vi "FT_Write_String_Data_64bit.vi"(4 "error in (no error)":errorcluster, 6 "Buffer":string, 7 "Handle":u64) -> (0 "error out":errorcluster, 1 "FT_Status":u32(ring) items=["FT_OK", "FT_INVALID_HANDLE", "FT_DEVICE_NOT_FOUND", "FT_DEVICE_NOT_OPENED", "FT_IO_ERROR", "FT_INSUFFICIENT_RESOURCES", "FT_INVALID_PARAMETER", "FT_INVALID_BAUD_RATE", "FT_DEVICE_NOT_OPENED_FOR_ERASE", "FT_DEVICE_NOT_OPENED_FOR_WRITE", "FT_FAILED_TO_WRITE_DEVICE", "FT_EEPROM_READ_FAILED", "FT_EEPROM_WRITE_FAILED", "FT_EEPROM_ERASE_FAILED", "FT_EEPROM_NOT_PRESENT", "FT_EEPROM_NOT_PROGRAMMED", "FT_INVALID_ARGS", "FT_NOT_SUPPORTED", "FT_OTHER_ERROR"], 2 "Bytes Written":u32, 3 "Handle out":u64)   [LabVIEW 2019]
uses:
  FTD2XX.dll
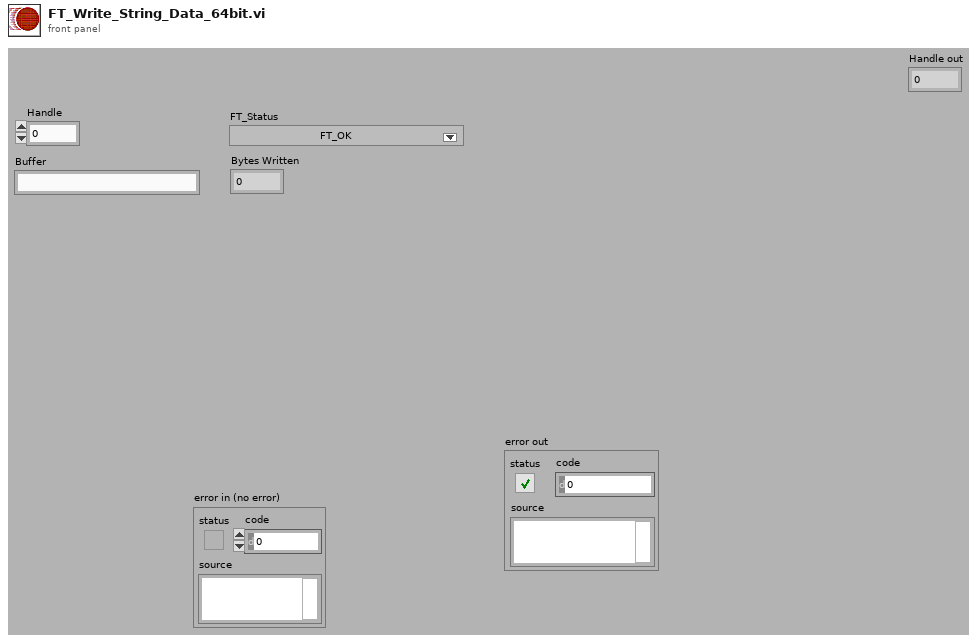
[diagram p1: front panel]
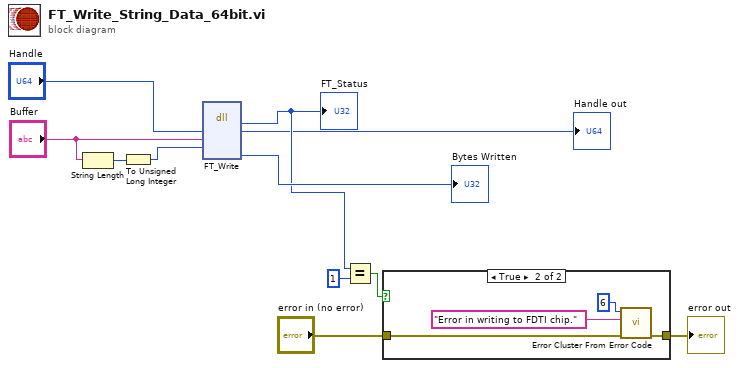
[diagram p0: block diagram]
diagram:
  n1 = String Length(string="Buffer") -> (length=w8:i32)
  n2 = To Unsigned Long Integer(number=w8) -> (unsigned 32bit integer=w7:u32)
  n3 = dll-call lib="FTD2XX.dll" fn="FT_Write"("Handle"="Handle", "Buffer"="Buffer", "BytesToWrite"=w7) -> ("FT_Status"=w2:u32, "Handle"=→"Handle out":u64, "BytesWritten"=→"Bytes Written":u32)  [unwired: 6 in, 2 out]
  "FT_Status" <- w2
  n4 = Equal?(x=w2, y=u32 1) -> (x = y?=w6:bool)
  n5 = case shown="True" w6 {
    tunnel: [w12 w15] -> w3
    tunnel: "error in (no error)" -> [w12 w14]
    frame False {
    }
    frame True {
      n6 = call <vilib>:"Error Cluster From Error Code.vi"("error in (no error)"=w14, "error message (\"\")"="Error in writing to FDTI chip." ("error message (\"\")"), "error code (0)"=6) -> ("error out"=w15:errorcluster)  [unwired: 6 in]
    }
  }
  "error out" <- w3
